vi "Clear.vi"(8 "error in (no error)":errorcluster, 11 "Mock In":refnum<class "Responsive Mock.lvclass">) -> (0 "error out":errorcluster)   [LabVIEW 2020, in "Responsive Mock.lvclass"]
doc: "Template method which should be overriden to clear anything which has been initialized during the lifecycle of the mock class. \nThis VI is called when the mock is verified, which marks the end of its lifecycle."
uses:
  Responsive Mock.lvclass
  Responsive Mock.lvclass/Responsive Mock.ctl
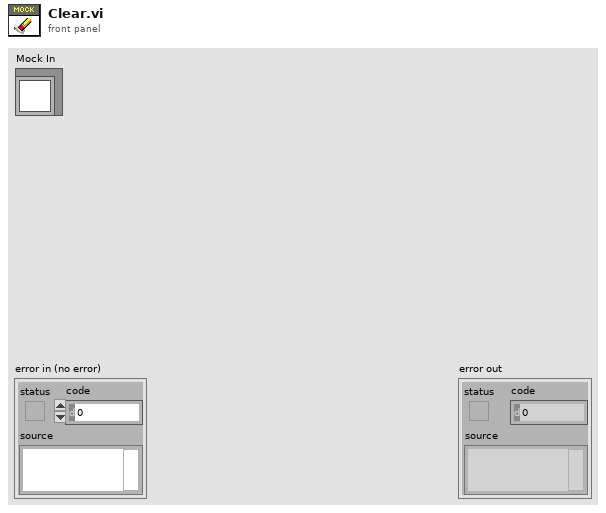
[diagram p1: front panel]
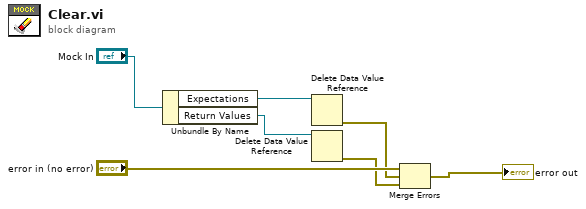
[diagram p0: block diagram]
diagram:
  n1 = Unbundle By Name("Mock In") -> ("Expectations"=w6:refnum<data-value>, "Return Values"=w2:refnum<data-value>)
  n2 = Delete Data Value Reference(data value reference=w6) -> (error out=w3:errorcluster)  [unwired: 1 in, 1 out]
  n3 = Delete Data Value Reference(data value reference=w2) -> (error out=w1:errorcluster)  [unwired: 1 in, 1 out]
  n4 = Merge Errors("error in (no error)", w3, w1) -> (→"error out":errorcluster)
